vi "Test.vi"() -> ()   [LabVIEW 2020, in "Library Instrument & Equipement.lvlib" / "Library DIO.lvlib"]
uses:
  Library DIO.lvlib
  Class DIO NI/Class DIO NI.lvclass
  C:/Users/ngarcin/OneDrive - Altyor/Standard TB/Class/DIO/Class DIO (Default)/Class DIO (Default).lvclass
panel:
  in  "stop 2":bool
  out "Value to Read":bool
  in  "stop":bool
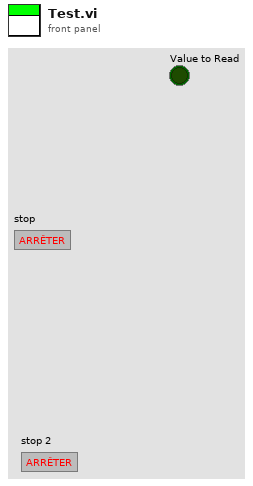
[diagram p1: front panel]
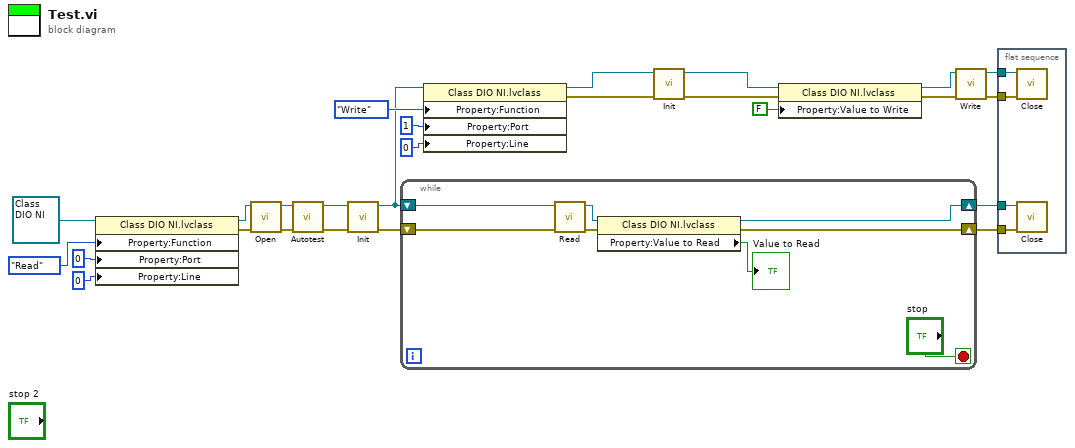
[diagram p0: block diagram]
diagram:
  n1 = property class="Class DIO NI.lvclass"(reference=refnum<class "Class DIO NI.lvclass"> refnum ("Library DIO.lvlib:Class DIO NI.lvclass"), "Property:Function"=enum16{"Write", "Read"}."Read" ("Function"), "Property:Port"=u8 0 ("Port"), "Property:Line"=u8 0 ("Line")) -> (reference out=w20:refnum<class "Class DIO NI.lvclass">, error out=w16:errorcluster)  [unwired: 1 in]
  n2 = call-dynamic "Open.vi"("error in (no error)"=w16, "Class DIO (Default) en entrée"=w20) -> ("error out"=w24:errorcluster, "Class DIO (Default) en sortie"=w26:refnum<class "Class DIO NI.lvclass">)  [unwired: 8 in]
  n3 = call-dynamic "Autotest.vi"("error in (no error)"=w24, "Class DIO (Default) en entrée"=w26) -> ("error out"=w23:errorcluster, "Class DIO (Default) en sortie"=w25:refnum<class "Class DIO NI.lvclass">)  [unwired: 7 in, 1 out]
  n4 = call-dynamic "Init.vi"("error in (no error)"=w23, "Class DIO (Default) en entrée"=w25) -> ("error out"=w22:errorcluster, "Class DIO (Default) en sortie"=w7:refnum<class "Class DIO NI.lvclass">)  [unwired: 8 in]
  n5 = while {
    shift-right: [w28] -> w2
    shift-left: w7 -> [w34]
    shift-right: [w27] -> w1
    shift-left: w22 -> [w33]
    stop <- "stop" stop-if-true
    n6 = call-dynamic "Read.vi"("error in (no error)"=w33, "Class DIO (Default) en entrée"=w34) -> ("error out"=w30:errorcluster, "Class DIO (Default) en sortie"=w32:refnum<class "Class DIO NI.lvclass">)  [unwired: 8 in]
    n7 = property class="Class DIO NI.lvclass"(reference=w32, error in=w30) -> (reference out=w28:refnum<class "Class DIO NI.lvclass">, error out=w27:errorcluster, "Property:Value to Read"=→"Value to Read":bool)
  }
  n8 = property class="Class DIO NI.lvclass"(reference=w7, "Property:Function"=enum16{"Write", "Read"}."Write" ("Function"), "Property:Port"=u8 1 ("Port"), "Property:Line"=u8 0 ("Line")) -> (reference out=w6:refnum<class "Class DIO NI.lvclass">, error out=w5:errorcluster)  [unwired: 1 in]
  n9 = call-dynamic "Init.vi"("error in (no error)"=w5, "Class DIO (Default) en entrée"=w6) -> ("error out"=w10:errorcluster, "Class DIO (Default) en sortie"=w12:refnum<class "Class DIO NI.lvclass">)  [unwired: 8 in]
  n10 = property class="Class DIO NI.lvclass"(reference=w12, error in=w10, "Property:Value to Write"=FALSE ("Value to Write")) -> (reference out=w11:refnum<class "Class DIO NI.lvclass">, error out=w9:errorcluster)
  n11 = call-dynamic "Write.vi"("error in (no error)"=w9, "Class DIO (Default) en entrée"=w11) -> ("error out"=w3:errorcluster, "Class DIO (Default) en sortie"=w4:refnum<class "Class DIO NI.lvclass">)  [unwired: 8 in]
  n12 = flat-sequence {
    tunnel: w1 -> [w38]
    tunnel: w2 -> [w37]
    tunnel: w3 -> [w36]
    tunnel: w4 -> [w35]
    frame #0 {
      n13 = call-dynamic "Close.vi"("error in (no error)"=w36, "Class DIO (Default) en entrée"=w35) -> ()  [unwired: 8 in, 2 out]
      n14 = call-dynamic "Close.vi"("error in (no error)"=w38, "Class DIO (Default) en entrée"=w37) -> ()  [unwired: 8 in, 2 out]
    }
  }
